vi "棋盘格标定.vi"() -> ()   [LabVIEW 2014]
uses:
  <vilib>/vision/Calibration.llb/Calibration Reference Points.ctl
  <vilib>/Utility/error.llb/DialogType.ctl
  <vilib>/vision/Calibration.llb/Distortion Model.ctl
  <vilib>/vision/Calibration.llb/Distortion Model Types.ctl
  <vilib>/vision/NI_Vision_Development_Module.lvlib
panel:
  in  "布尔":bool
  out "ROI Descriptor":T1 {"Contours"."Type" items=["No Selection", "Point", "Line", "Rectangle", "Oval", "Polygon", "Freehand Region", "Annulus", "Unused2", "Unused3", "Broken Line", "Freehand Line", "Rotated Rectangle"]}
  in  "停止按钮":bool
  in  "删除按钮":bool
  in  "刷新按钮":bool
  in  "角点检测参数设置":T2={"角点检测算法选择"=0, "Kernel 尺寸"=3, "最小的角点强度"=20.0} {"角点检测算法选择" items=["Harris Corner", "Shi-Tomasi Corner"]; "Kernel 尺寸" min=3 max=9 step=2}
  in  "进行图像标定":bool
  out "标定完成":bool
  out "Location":cluster{"X":sgl, "Y":sgl}
  in  "X轴方向间距":i32
  in  "Y轴方向间距":i32
  in  "Reference Points":T3
  in  "单位选择":u16(ring) items=["Undefined", "Angstr", "Micrometer", "Millimeter", "Centimeter", "Meter", "Kilometer", "Microinch", "Inch", "Feet", "Nautical miles", "Standardmiles", "Steps"]
  out "角点图":T5(plugin-control)
  out "图像尺寸":cluster{"X":u32, "Y":u32}
  # "棋盘格标定"
  # "说明：\n    请保证棋盘格每行的角\n点数一样，且每一列的角\n点数也一样；对于多余的\n角点，单击【奇异角点删\n除】进行多余的角点的删\n除。"
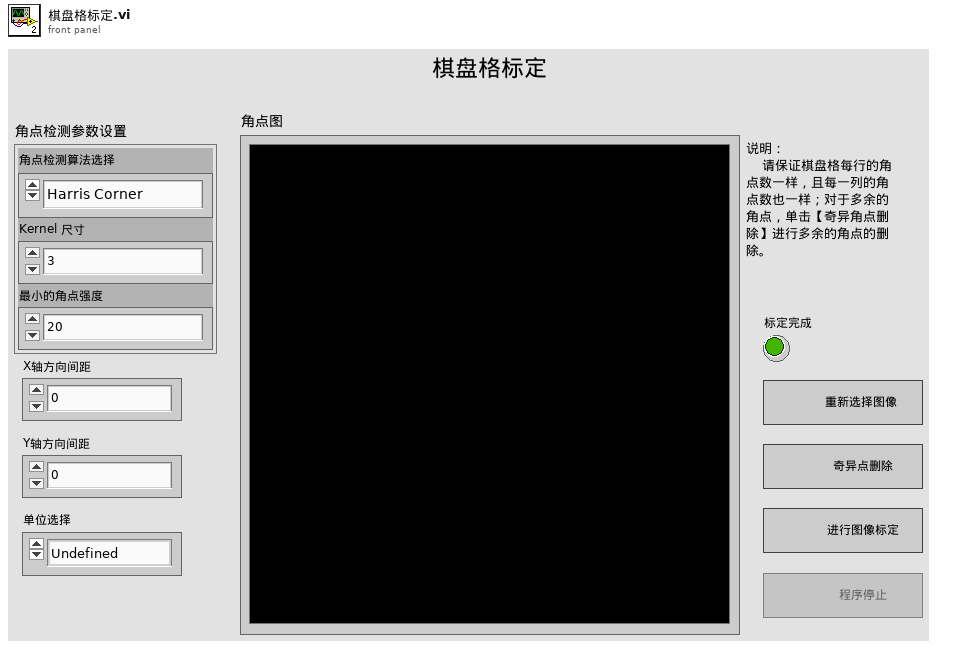
[diagram p1: front panel]
types:
  T1 = typedef "ROI Descriptor" = cluster{"Global Rectangle":i32[], "Contours":cluster{"ID":enum32{"External", "Internal"}, "Type":u32, "Coordinates":i32[]}[]}
  T2 = cluster{"角点检测算法选择":u16, "Kernel 尺寸":i32, "最小的角点强度":dbl}
  T3 = typedef "Calibration Reference Points.ctl" = cluster{"Pixel Coordinates":cluster{"X":dbl, "Y":dbl}[], "Real World Coordinates":cluster{"X":dbl, "Y":dbl}[], "Unit":T4, "Image Size":cluster{"X":u32, "Y":u32}}
  T4 = typedef "Image Unit" = enum32{"Undefined", "Angström", "Micrometer", "Millimeter", "Centimeter", "Meter", "Kilometer", "Microinch", "Inch", "Feet", "Nautical miles", "Standard miles", "Steps"}
  T5 = typedef "IMAQ Image.ctl" = refnum<image>
  T6 = enum8{"Enabled", "Disabled", "Disabled and Grayed Out"}
  T7 = typedef "Image Type" = u32
  T8 = typedef "IMAQ Rectangle" = cluster{"Left":i32, "Top":i32, "Right":i32, "Bottom":i32, "Rotation":dbl}
  T9 = enum32{"Invalid", "Standard", "Closed", "Hidden", "Minimized", "Maximized"}
  T10 = typedef "DialogType.ctl" = u16
  T11 = typedef "Distortion Model.ctl" = cluster{"Distortion Model":T12, "Polynomial Model Setup":cluster{"Radial Coefficient":u32, "Tangential Coefficients ":bool}}
  T12 = typedef "Distortion Model Types.ctl" = i32
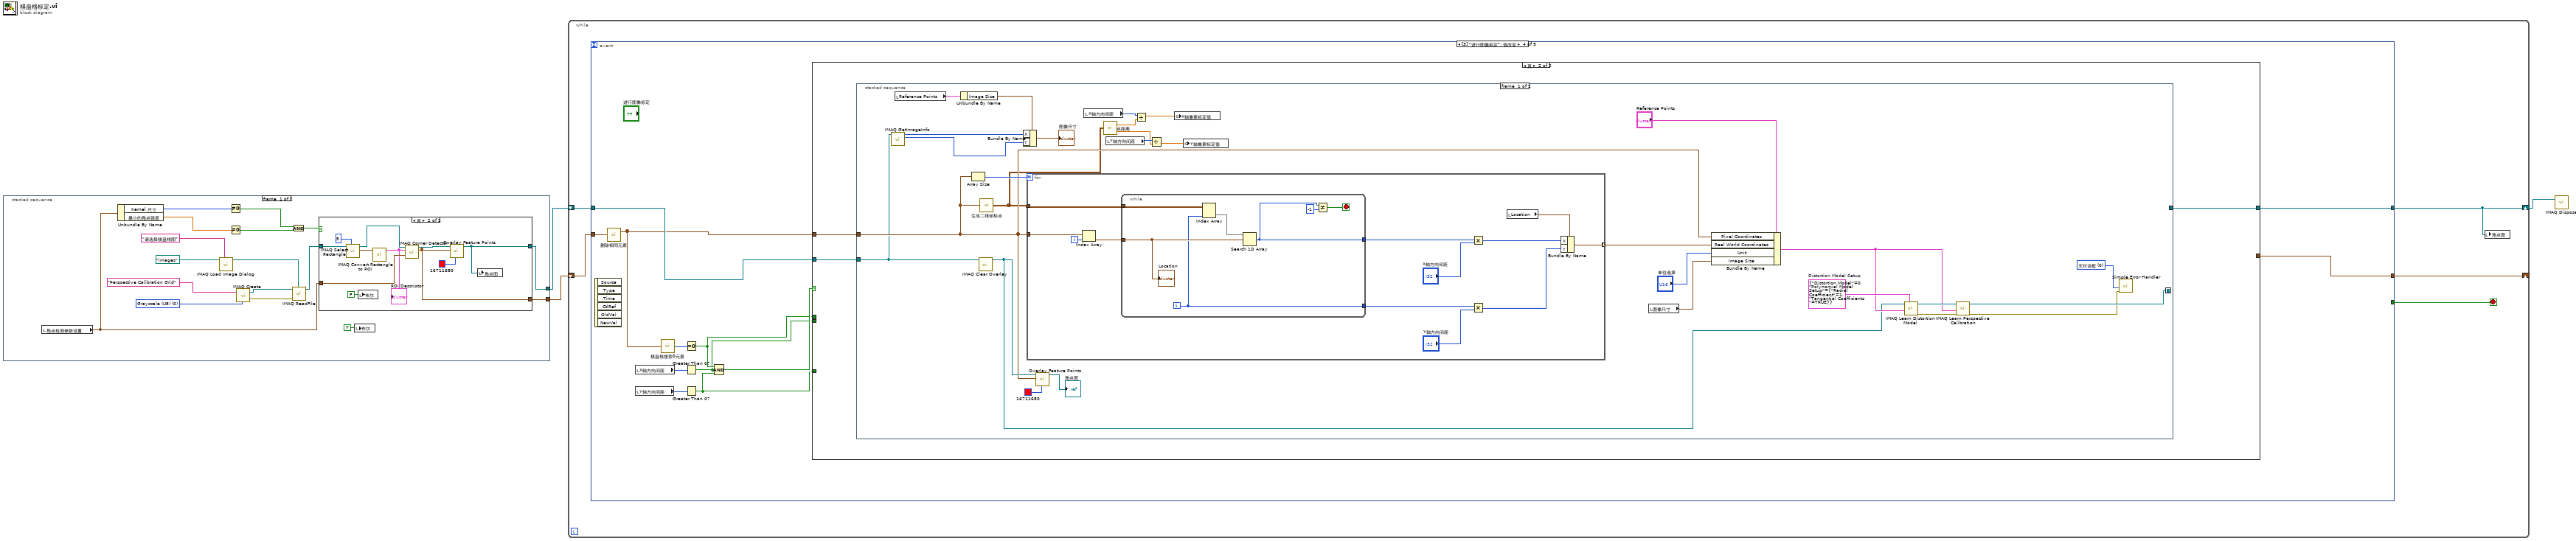
[diagram p0: block diagram]
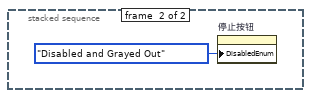
[diagram p3: hidden frame]
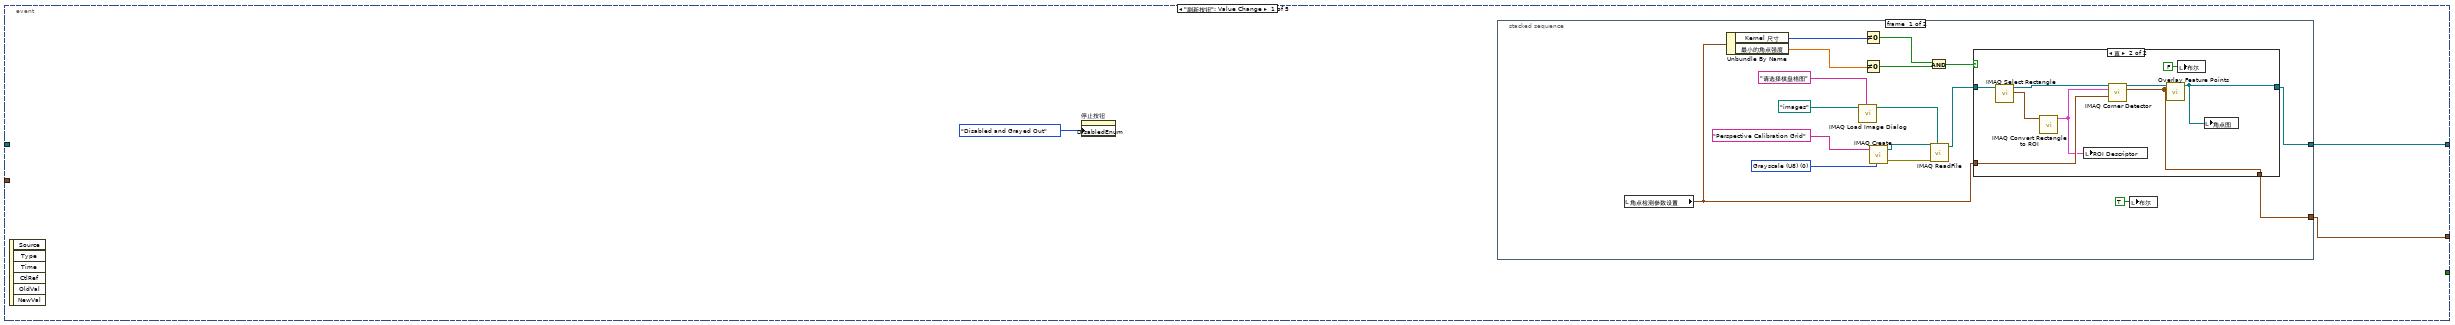
[diagram p4: hidden frame]
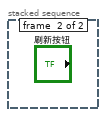
[diagram p6: hidden frame]
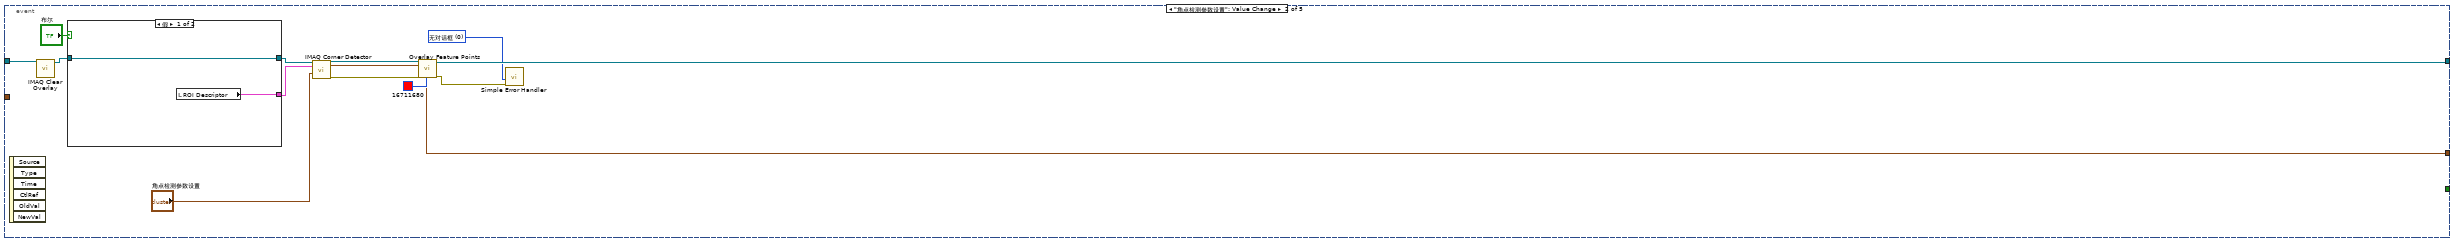
[diagram p7: hidden frame]
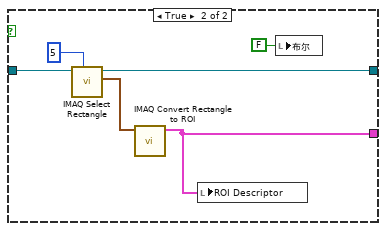
[diagram p8: hidden frame]
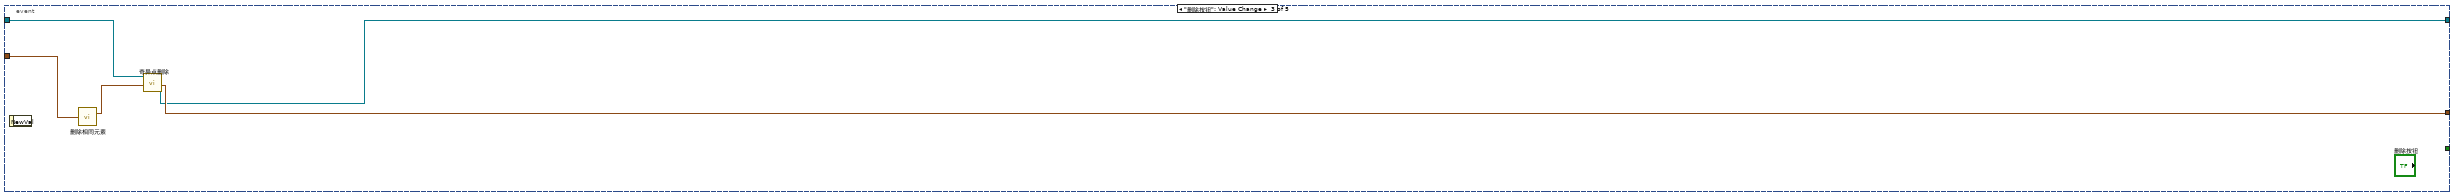
[diagram p9: hidden frame]
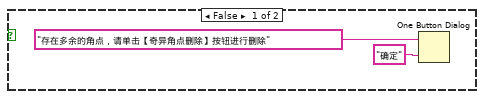
[diagram p11: hidden frame]
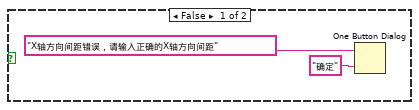
[diagram p13: hidden frame]
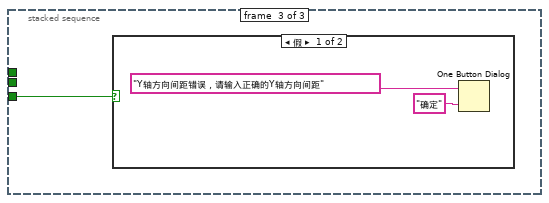
[diagram p14: hidden frame]
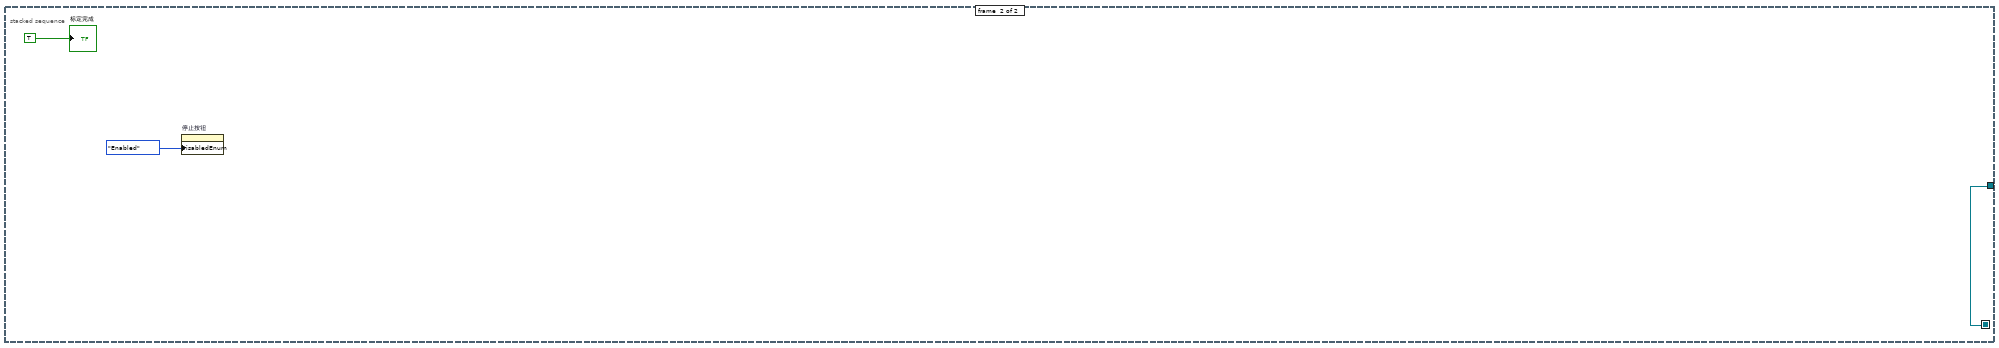
[diagram p16: hidden frame]
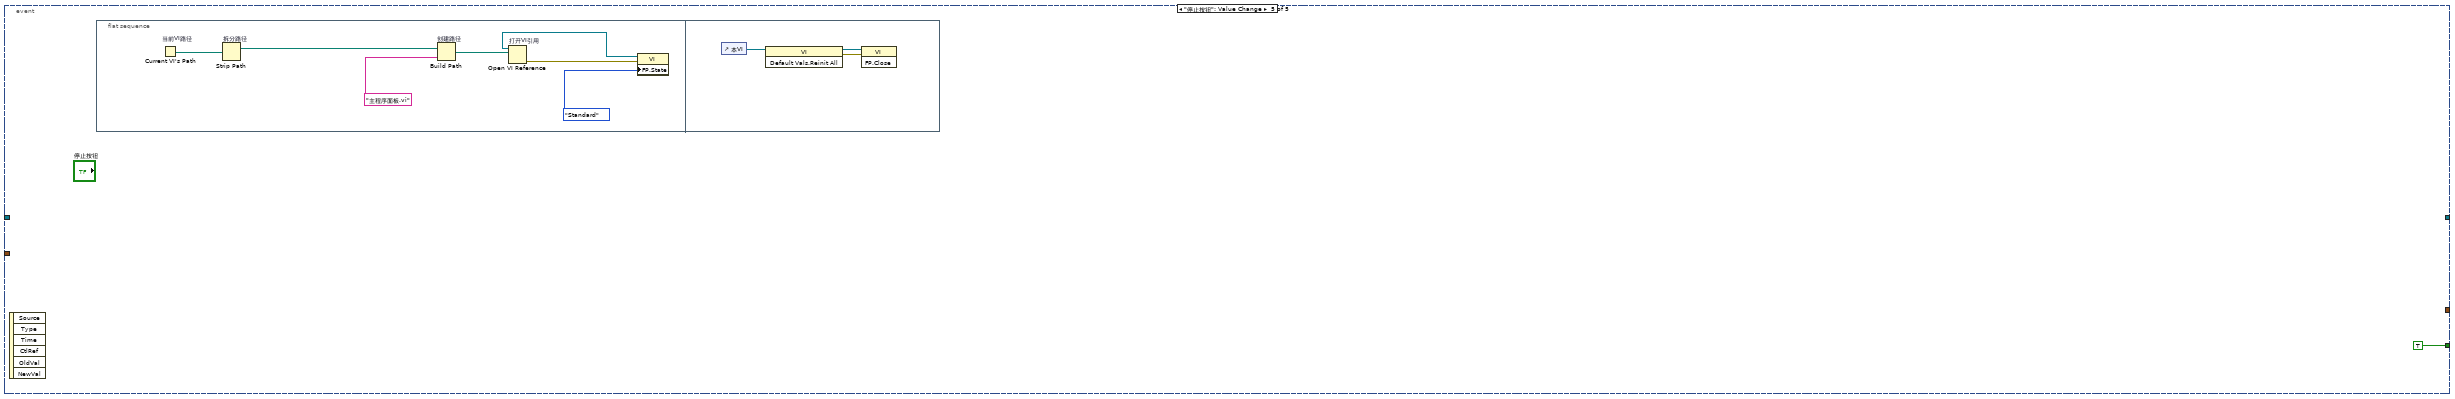
[diagram p17: hidden frame]
diagram:
  n1 = stacked-sequence {
    tunnel: [w6 _] -> w3
    tunnel: [w5 _] -> w1
    frame #0 {
      w7 = T7 0 items=["Grayscale (U8)", "Grayscale (I16)", "Grayscale (SGL)", "Complex (CSG)", "RGB (U32)", "HSL (U32)", "RGB (U64)", "Grayscale (U16)"] ("Image Type")
      n2 = local read "角点检测参数设置"() -> (w15:T2)
      n3 = Unbundle By Name(w15) -> ("Kernel 尺寸"=w16:i32, "最小的角点强度"=w17:dbl)
      n4 = call "IMAQ Load Image Dialog"("Prompt"="请选择棋盘格图" ("prompt"), "Start Path"=path "images") -> ("Path"=w9:path)  [unwired: 7 in, 2 out]
      n5 = Not Equal To 0?(x=w16) -> (x != 0?=w18:bool)
      n6 = Not Equal To 0?(x=w17) -> (x != 0?=w19:bool)
      n7 = call "IMAQ Create"("Image Name"="Perspective Calibration Grid", "Image Type"=w7) -> ("New Image"=w12:T5, "error out"=w11:errorcluster)  [unwired: 2 in, 1 out]
      n8 = And(x=w18, y=w19) -> (x .and. y?=w20:bool)
      n9 = call "IMAQ ReadFile"("File Path"=w9, "error in (no error)"=w11, "Image"=w12) -> ("Image Out"=w14:T5)  [unwired: 2 in, 6 out]
      n10 = case shown="真" w20 {
        tunnel: w15 -> [_ w32]
        tunnel: [w21 w30] -> w6
        tunnel: w14 -> [w21 w24]
        tunnel: [_ w28] -> w5
        frame False {
        }
        frame True {
          n11 = call "IMAQ Select Rectangle"("Window Number (0...15)"=5, "Image In"=w24) -> ("Rectangle"=w25:T8, "Image Out (duplicate)"=w27:T5)  [unwired: 6 in, 2 out]
          n12 = local write "布尔"(FALSE ("布尔")) -> ()
          n13 = call "IMAQ Convert Rectangle to ROI"("Rectangle"=w25) -> ("ROI Descriptor"=w26:T1)  [unwired: 8 in, 1 out]
          "ROI Descriptor" <- w26
          n14 = call "IMAQ Corner Detector"("Image"=w27, "ROI Descriptor"=w26, "Corner Options"=w32) -> ("Image (duplicate)"=w31:T5, "Corner Point Coordinates"=w28:cluster{"X":sgl, "Y":sgl}[])  [unwired: 7 in, 4 out]
          n15 = call "Overlay Feature Points.vi"("Color"=u32 16711680, "Feature Points"=w28, "Image"=w31) -> ("Image Out"=w30:T5)  [unwired: 7 in, 1 out]
          n16 = local write "角点图"(w30) -> ()
        }
      }
      n17 = local write "布尔"(TRUE ("布尔")) -> ()
    }
    frame #1 {
      n18 = property on="停止按钮" class="Bool"("DisabledEnum"=T6."Disabled and Grayed Out" ("禁用")) -> ()  [unwired: 2 in, 2 out]
    }
  }
  n19 = while {
    shift-right: [w34] -> w2
    shift-left: w3 -> [w36]
    shift-right: [w38] -> _
    shift-left: w1 -> [w37]
    stop <- w35 stop-if-true
    n20 = event shown="[3] \"进行图像标定\": 值改变" {
      selector: _ -> [_ _ _ _ _]
      dyn-events: _ -> [_ _ _ _ _]
      timeout: _ -> [_ _ _ _ _]
      tunnel: [w41 w78 w90 w104 _] -> w34
      tunnel: [w40 w76 w92 w105 _] -> w38
      tunnel: w37 -> [_ _ w94 w103 _]
      tunnel: w36 -> [_ w79 w91 w106 _]
      tunnel: [_ _ _ _ TRUE] -> w35
      event "刷新按钮": Value Change {
        n21 = event-data() -> ()  [unwired: 1 in, 6 out]
        n22 = property on="停止按钮" class="Bool"("DisabledEnum"=T6."Disabled and Grayed Out" ("禁用")) -> ()  [unwired: 2 in, 2 out]
        n23 = stacked-sequence {
          tunnel: [w44 _] -> w41
          tunnel: [w43 _] -> w40
          frame #0 {
            w45 = T7 0 items=["Grayscale (U8)", "Grayscale (I16)", "Grayscale (SGL)", "Complex (CSG)", "RGB (U32)", "HSL (U32)", "RGB (U64)", "Grayscale (U16)"] ("Image Type")
            n24 = local read "角点检测参数设置"() -> (w53:T2)
            n25 = Unbundle By Name(w53) -> ("Kernel 尺寸"=w54:i32, "最小的角点强度"=w55:dbl)
            n26 = call "IMAQ Load Image Dialog"("Prompt"="请选择棋盘格图" ("prompt"), "Start Path"=path "images") -> ("Path"=w47:path)  [unwired: 7 in, 2 out]
            n27 = Not Equal To 0?(x=w54) -> (x != 0?=w56:bool)
            n28 = Not Equal To 0?(x=w55) -> (x != 0?=w57:bool)
            n29 = call "IMAQ Create"("Image Name"="Perspective Calibration Grid", "Image Type"=w45) -> ("New Image"=w50:T5, "error out"=w49:errorcluster)  [unwired: 2 in, 1 out]
            n30 = And(x=w56, y=w57) -> (x .and. y?=w58:bool)
            n31 = call "IMAQ ReadFile"("File Path"=w47, "error in (no error)"=w49, "Image"=w50) -> ("Image Out"=w52:T5)  [unwired: 2 in, 6 out]
            n32 = case shown="真" w58 {
              tunnel: w53 -> [_ w68]
              tunnel: [w59 w66] -> w44
              tunnel: w52 -> [w59 w64]
              tunnel: [_ w65] -> w43
              frame False {
              }
              frame True {
                n33 = call "IMAQ Select Rectangle"("Image In"=w64) -> ("Rectangle"=w62:T8, "Image Out (duplicate)"=w63:T5)  [unwired: 7 in, 2 out]
                n34 = call "IMAQ Convert Rectangle to ROI"("Rectangle"=w62) -> ("ROI Descriptor"=w61:T1)  [unwired: 8 in, 1 out]
                n35 = local write "ROI Descriptor"(w61) -> ()
                n36 = call "IMAQ Corner Detector"("Image"=w63, "ROI Descriptor"=w61, "Corner Options"=w68) -> ("Image (duplicate)"=w67:T5, "Corner Point Coordinates"=w65:cluster{"X":sgl, "Y":sgl}[])  [unwired: 7 in, 4 out]
                n37 = call "Overlay Feature Points.vi"("Feature Points"=w65, "Image"=w67) -> ("Image Out"=w66:T5)  [unwired: 8 in, 1 out]
                n38 = local write "布尔"(FALSE ("布尔")) -> ()
                n39 = local write "角点图"(w66) -> ()
              }
            }
            n40 = local write "布尔"(TRUE ("布尔")) -> ()
          }
          frame #1 {
          }
        }
      }
      event "角点检测参数设置": Value Change {
        w73 = T10 0 items=["无对话框", "确定信息", "继续或停止信息", "确定信息＋警告", "继续/停止+警告"] ("type of dialog (OK msg:1)")
        n41 = event-data() -> ()  [unwired: 1 in, 6 out]
        n42 = call "IMAQ Clear Overlay"("Image"=w79) -> ("Image Out"=w72:T5)  [unwired: 9 in, 1 out]
        n43 = case shown="假" "布尔" {
          tunnel: w72 -> [w83 w89]
          tunnel: [w83 w88] -> w71
          tunnel: [w82 w85] -> w70
          frame False {
            n44 = local read "ROI Descriptor"() -> (w82:T1)
          }
          frame True {
            n45 = call "IMAQ Select Rectangle"("Window Number (0...15)"=5, "Image In"=w89) -> ("Rectangle"=w87:T8, "Image Out (duplicate)"=w88:T5)  [unwired: 6 in, 2 out]
            n46 = call "IMAQ Convert Rectangle to ROI"("Rectangle"=w87) -> ("ROI Descriptor"=w85:T1)  [unwired: 8 in, 1 out]
            n47 = local write "ROI Descriptor"(w85) -> ()
            n48 = local write "布尔"(FALSE ("布尔")) -> ()
          }
        }
        n49 = call "IMAQ Corner Detector"("Image"=w71, "ROI Descriptor"=w70, "Corner Options"="角点检测参数设置") -> ("Image (duplicate)"=w77:T5, "Corner Point Coordinates"=w76:cluster{"X":sgl, "Y":sgl}[], "error out"=w75:errorcluster)  [unwired: 7 in, 3 out]
        n50 = call "Overlay Feature Points.vi"("Color"=u32 16711680, "error in"=w75, "Feature Points"=w76, "Image"=w77) -> ("error out"=w74:errorcluster, "Image Out"=w78:T5)  [unwired: 6 in]
        n51 = call <vilib>:"Simple Error Handler.vi"("type of dialog (OK msg:1)"=w73, "error in (no error)"=w74) -> ()  [unwired: 3 in, 5 out]
      }
      event "删除按钮": Value Change {
        n52 = event-data() -> ()  [unwired: 1 in, 1 out]
        n53 = call "删除相同元素.vi"("输入"=w94) -> ("输出"=w93:cluster{"X":sgl, "Y":sgl}[])  [unwired: 1 out]
        n54 = call "奇异点删除.vi"("原始角点坐标"=w93, "Image In"=w91) -> ("原始角点坐标 2"=w92:cluster{"X":sgl, "Y":sgl}[], "角点图"=w90:T5)  [unwired: 6 in]
      }
      event "进行图像标定": Value Change {
        n55 = event-data() -> ()  [unwired: 1 in, 6 out]
        n56 = call "删除相同元素.vi"("输入"=w103) -> ("输出"=w102:cluster{"X":sgl, "Y":sgl}[])  [unwired: 1 out]
        n57 = local read "X轴方向间距"() -> (w101:i32)
        n58 = local read "Y轴方向间距"() -> (w100:i32)
        n59 = call "棋盘格搜索0元素.vi"("无序一维坐标点"=w102) -> ("数值输入控件"=w99:i32)
        n60 = Equal To 0?(x=w99) -> (x = 0?=w97:bool)
        n61 = Greater Than 0?(x=w101) -> (x > 0?=w96:bool)
        n62 = Greater Than 0?(x=w100) -> (x > 0?=w95:bool)
        n63 = Compound Arithmetic op=AND(w97, w96, w95) -> (w98:bool)
        n64 = case shown="真" w98 {
          tunnel: w102 -> [w111 w123]
          tunnel: w106 -> [w110 w122]
          tunnel: [w111 _] -> w105
          tunnel: [w110 w121] -> w104
          tunnel: w97 -> [w109 _]
          tunnel: w96 -> [w108 _]
          tunnel: w95 -> [w107 _]
          frame False {
            n65 = stacked-sequence {
              tunnel: w109 -> [w112 _ _]
              tunnel: w108 -> [_ w115 _]
              tunnel: w107 -> [_ _ w118]
              frame #0 {
                n66 = case shown="真" w112 {
                  frame False {
                    n67 = One Button Dialog(message="存在多余的角点，请单击【奇异角点删除】按钮进行删除" ("消息"), button name ("OK")="确定" ("按钮名称（“确定”）")) -> ()  [unwired: 1 out]
                  }
                  frame True {
                  }
                }
              }
              frame #1 {
                n68 = case shown="真" w115 {
                  frame False {
                    n69 = One Button Dialog(message="X轴方向间距错误，请输入正确的X轴方向间距" ("消息"), button name ("OK")="确定" ("按钮名称（“确定”）")) -> ()  [unwired: 1 out]
                  }
                  frame True {
                  }
                }
              }
              frame #2 {
                n70 = case shown="假" w118 {
                  frame False {
                    n71 = One Button Dialog(message="Y轴方向间距错误，请输入正确的Y轴方向间距" ("消息"), button name ("OK")="确定" ("按钮名称（“确定”）")) -> ()  [unwired: 1 out]
                  }
                  frame True {
                  }
                }
              }
            }
          }
          frame True {
            n72 = stacked-sequence {
              seq-local: [w125 _] -> [_ w174]
              tunnel: w123 -> [w140 _]
              tunnel: w122 -> [w133 _]
              tunnel: [_ w174] -> w121
              frame #0 {
                w148 = T10 0 items=["无对话框", "确定信息", "继续或停止信息", "确定信息＋警告", "继续/停止+警告"] ("type of dialog (OK msg:1)")
                w150 = T11 {"Distortion Model"=0, "Polynomial Model Setup"={"Radial Coefficient"=1, "Tangential Coefficients "=TRUE}}  # Distortion Model Setup
                n73 = call "IMAQ GetImageInfo"("Image"=w133) -> ("Y Resolution"=w137:i32, "X Resolution"=w138:i32)  [unwired: 3 in, 6 out]
                n74 = local read "Reference Points"() -> (w136:T3)
                n75 = Unbundle By Name(w136) -> ("Image Size"=w135:cluster{"X":u32, "Y":u32})
                n76 = Array Size(array=w140) -> (size(s)=w152:i32)
                n77 = call "IMAQ Clear Overlay"("Image"=w133) -> ("Image Out"=w139:T5)  [unwired: 9 in, 1 out]
                n78 = call "生成二维坐标点.vi"("输入无序一维坐标点"=w140) -> ("输出有序二维坐标点"=w132:cluster{"X":sgl, "Y":sgl}[][])
                n79 = Bundle By Name(cluster=w135, "X"=w138, "Y"=w137) -> (→"图像尺寸":cluster{"X":u32, "Y":u32})
                n80 = for {
                  N: w152 -> [_]
                  tunnel: w132 -> [w163]
                  tunnel: w140 -> [w153]
                  tunnel: [w154] -> w145 mode=indexing
                  i -> [w164]
                  n81 = Index Array(array=w153, index=w164) -> (element=w162:cluster{"X":sgl, "Y":sgl})
                  n82 = while {
                    tunnel: w163 -> [w170]
                    tunnel: w162 -> [w171]
                    tunnel: [w166] -> w158
                    tunnel: [w167] -> w159
                    i -> [w166]
                    stop <- w168 stop-if-true
                    n83 = Index Array(array=w170, index (col)=w166) -> (element=w165:cluster{"X":sgl, "Y":sgl}[])  [unwired: 1 in]
                    n84 = Search 1D Array(1D array=w165, element=w171) -> (index of element=w167:i32)  [unwired: 1 in]
                    n85 = Not Equal?(x=w167, y=-1) -> (x != y?=w168:bool)
                    "Location" <- w171
                  }
                  n86 = Multiply(x=w159, y="X轴方向间距") -> (x*y=w157:i32)
                  n87 = Multiply(x=w158, y="Y轴方向间距") -> (x*y=w156:i32)
                  n88 = local read "Location"() -> (w155:cluster{"X":sgl, "Y":sgl})
                  n89 = Bundle By Name(cluster=w155, "X"=w157, "Y"=w156) -> (w154:cluster{"X":sgl, "Y":sgl})
                }
                n90 = call "Overlay Feature Points.vi"("Color"=u32 16711680, "Feature Points"=w140, "Image"=w139) -> ("Image Out"=→"角点图":T5)  [unwired: 7 in, 1 out]
                n91 = local read "X轴方向间距"() -> (w131:i32)
                n92 = call "点距离.vi"("二维点阵"=w132) -> ("X间距"=w130:sgl, "Y间距"=w128:sgl)
                n93 = local read "Y轴方向间距"() -> (w129:i32)
                n94 = Divide(x=w131, y=w130) -> (x/y=w127:sgl)
                n95 = Divide(x=w129, y=w128) -> (x/y=w126:sgl)
                n96 = global write "全局变量.vi" "X轴像素标定值"(w127) -> ()
                n97 = global write "全局变量.vi" "Y轴像素标定值"(w126) -> ()
                n98 = local read "图像尺寸"() -> (w143:cluster{"X":u32, "Y":u32})
                n99 = Bundle By Name(cluster="Reference Points", "Pixel Coordinates"=w140, "Real World Coordinates"=w145, "Unit"="单位选择", "Image Size"=w143) -> (w146:T3)
                n100 = call "IMAQ Learn Distortion Model"("Distortion Model Setup"=w150, "Reference Points"=w146, "Calibration Template Image"=w139) -> ("error out"=w149:errorcluster, "Calibration Template Image Out"=w151:T5)  [unwired: 3 in, 4 out]
                n101 = call "IMAQ Learn Perspective Calibration"("error in (no error)"=w149, "Reference Points"=w146, "Calibration Template Image"=w151) -> ("error out"=w124:errorcluster, "Calibration Template Image Out"=w125:T5)  [unwired: 1 in, 6 out]
                n102 = call <vilib>:"Simple Error Handler.vi"("type of dialog (OK msg:1)"=w148, "error in (no error)"=w124) -> ()  [unwired: 3 in, 5 out]
              }
              frame #1 {
                n103 = property on="停止按钮" class="Bool"("DisabledEnum"=T6."Enabled" ("禁用")) -> ()  [unwired: 2 in, 2 out]
                "标定完成" <- TRUE ("标定完成")
              }
            }
          }
        }
      }
      event "停止按钮": Value Change {
        n104 = event-data() -> ()  [unwired: 1 in, 6 out]
        n105 = flat-sequence {
          frame #0 {
            n106 = Current VI's Path "当前VI路径"() -> (path=w180:path)
            n107 = Strip Path "拆分路径"(path=w180) -> (stripped path=w182:path)  [unwired: 1 out]
            n108 = Build Path "创建路径"(base path=w182, name or relative path="主程序面板.vi" ("名称或相对路径")) -> (appended path=w181:path)
            n109 = Open VI Reference "打开VI引用"(vi path=w181) -> (vi reference=w179:refnum<vi>, error out=w178:errorcluster)  [unwired: 5 in]
            n110 = property class="VI"(reference=w179, error in=w178, "FP.State"=T9."Standard" ("前面板窗口:状态")) -> ()  [unwired: 2 out]
          }
          frame #1 {
            n111 = control-ref of="本VI"() -> (w183:refnum<vi>)
            n112 = invoke class="VI" method="Default Vals.Reinit All"(reference=w183) -> (reference out=w184:refnum<vi>, error out=w185:errorcluster)  [unwired: 2 in, 1 out]
            n113 = invoke class="VI" method="FP.Close"(reference=w184, error in=w185) -> ()  [unwired: 1 in, 3 out]
          }
        }
      }
    }
    n114 = local write "角点图"(w34) -> ()
  }
  n115 = call "IMAQ Dispose"("Image"=w2) -> ()  [unwired: 5 in, 1 out]
